vi "ROI_positions_LOAD.vi"(2 "error in":errorcluster, 3 "XY positions":dbl[][](array[numeric])) -> (0 "error out":errorcluster, 1 "XY positions OUT":dbl[][](array[numeric]))   [LabVIEW 2015]
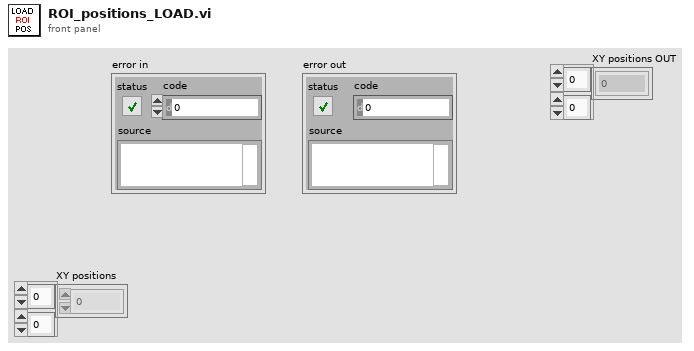
[diagram p1: front panel]
types:
  T1 = enum16{"open", "open or create", "create or replace", "create", "open (read-only)"}
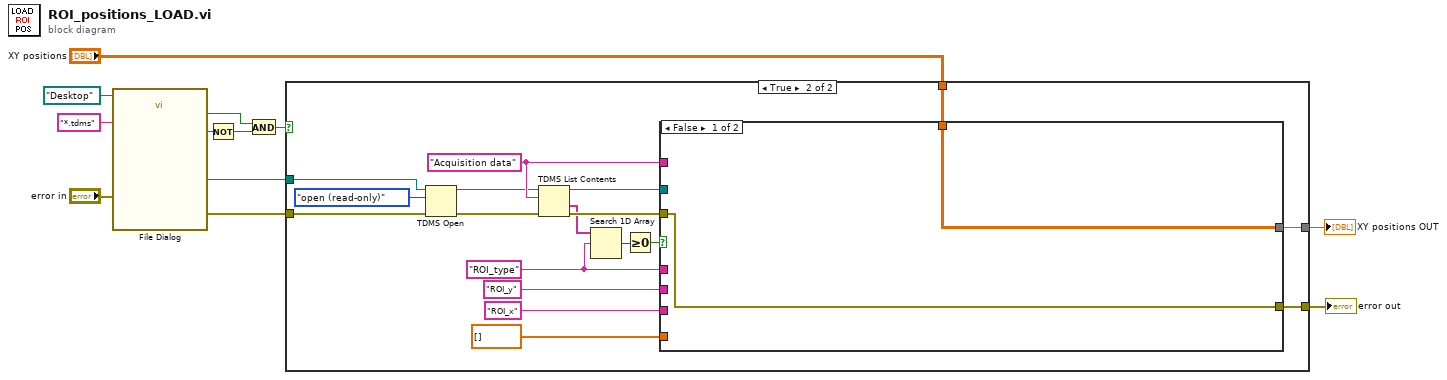
[diagram p0: block diagram]
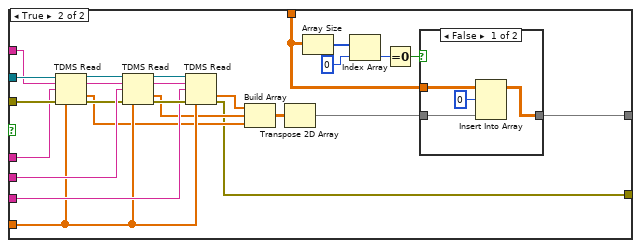
[diagram p3: hidden frame]
diagram:
  n1 = call "File Dialog"("start path"=path "Desktop", "error in"="error in", "pattern (all files)"="*.tdms") -> ("selected path"=w8:path, "exists"=w2:bool, "cancelled"=w9:bool, "error out"=w7:errorcluster)  [unwired: 9 in]
  n2 = Not(x=w9) -> (.not. x?=w1:bool)
  n3 = And(x=w2, y=w1) -> (x .and. y?=w6:bool)
  n4 = case shown="True" w6 {
    tunnel: w8 -> [_ w24]
    tunnel: w7 -> [w13 w22]
    tunnel: "XY positions" -> [w14 w20]
    tunnel: [w14 w19] -> w3
    tunnel: [w13 w18] -> w4
    frame False {
    }
    frame True {
      w16 = "ROI_type"
      w30 = "Acquisition data" ("group name in (Untitled)")
      n5 = TDMS Open(8:w22, 10:T1."open (read-only)" ("operation (0:open)"), 11:w24) -> (0:w25:errorcluster, 3:w17:refnum<k34>)  [unwired: 4 in]
      n6 = TDMS List Contents(4:w25, 6:w30, 7:w17) -> (0:w31:errorcluster, 1:w28:string[], 3:w29:refnum<k34>)  [unwired: 1 out]
      n7 = Search 1D Array(1D array=w28, element=w16) -> (index of element=w27:i32)  [unwired: 1 in]
      n8 = Greater Or Equal To 0?(x=w27) -> (x >= 0?=w32:bool)
      n9 = case shown="False" w32 {
        tunnel: "ROI_y" -> [_ w53]
        tunnel: w29 -> [_ w58]
        tunnel: w30 -> [_ w57]
        tunnel: w16 -> [_ w56]
        tunnel: w31 -> [w33 w59]
        tunnel: "ROI_x" -> [_ w48]
        tunnel: dbl[] [] -> [_ w47]
        tunnel: w20 -> [w34 w37]
        tunnel: [w34 w36] -> w19
        tunnel: [w33 w35] -> w18
        frame False {
        }
        frame True {
          n10 = TDMS Read(0:w58, 5:w57, 7:w56, 11:w59, 12:w47) -> (4:w55:refnum<k34>, 6:w54:string, 10:w43:dbl[], 15:w52:errorcluster)  [unwired: 3 in, 2 out]
          n11 = TDMS Read(0:w55, 5:w54, 7:w53, 11:w52, 12:w47) -> (4:w51:refnum<k34>, 6:w50:string, 10:w44:dbl[], 15:w49:errorcluster)  [unwired: 3 in, 2 out]
          n12 = TDMS Read(0:w51, 5:w50, 7:w48, 11:w49, 12:w47) -> (10:w45:dbl[], 15:w35:errorcluster)  [unwired: 3 in, 4 out]
          n13 = Build Array(w45, w44, w43) -> (w46:dbl[][])
          n14 = Transpose 2D Array(2D array=w46) -> (transposed array=w42:dbl[][])
          n15 = Array Size(array=w37) -> (size(s)=w41:i32[])
          n16 = Index Array(array=w41, index=0) -> (element=w39:i32)
          n17 = Equal To 0?(x=w39) -> (x = 0?=w38:bool)
          n18 = case shown="False" w38 {
            tunnel: w42 -> [w62 w64]
            tunnel: [w61 w64] -> w36
            tunnel: w37 -> [w60 _]
            frame False {
              n19 = Insert Into Array(array=w60, index (row)=0, new element=w62) -> (w61:dbl[][])  [unwired: 1 in]
            }
            frame True {
            }
          }
        }
      }
    }
  }
  "error out" <- w4
  "XY positions OUT" <- w3
